vi "Calc Formation Energy from Defect Cluster.vi"(4 "Dielectric Constant":dbl=11.0, 6 "Volume (A³)":dbl=7795.605843681768, 8 "Markov-Payne Correction":bool, 9 "Chemical Potential":dbl(slide)=0.5124378109452736 scale=0.0..1.0, 10 "Fermi Level (eV)":dbl=1.8, 11 "Defect Data":T1={"Defect Details"={"Defect Name"="Cd Frenkel anion", "Site Density"=1.0, "Reference Pure Structure Energy"=-159.32149, "N (Cd,Ideal - Cd,Defect)"=0, "N (Te,ideal - Te,defect)"=0}, "Charges and Energies"=[]}) -> (2 "Net Charge":i32, 3 "Formation Energy (eV)":dbl)   [LabVIEW 2010]
panel:
  out "Array":dbl[](array[numeric])
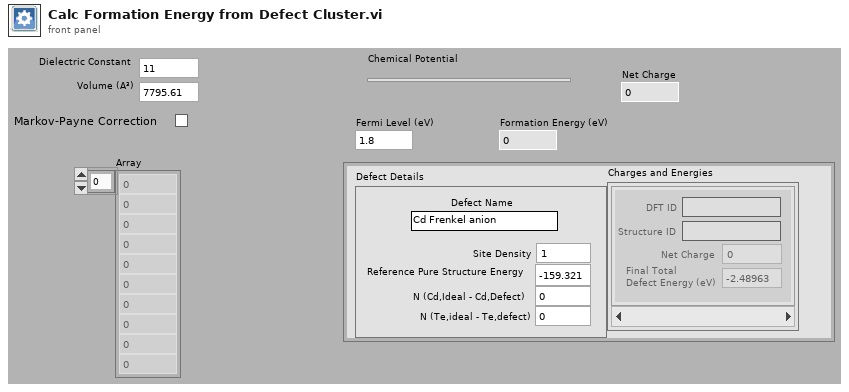
[diagram p1: front panel]
types:
  T1 = cluster{"Defect Details":cluster{"Defect Name":string, "Site Density":dbl, "Reference Pure Structure Energy":dbl, "N (Cd,Ideal - Cd,Defect)":i32, "N (Te,ideal - Te,defect)":i32}, "Charges and Energies":cluster{"DFT ID":string, "Structure ID":string, "Net Charge":i32, "Final Total \nDefect Energy (eV)":dbl}[]}
  T2 = cluster{"Defect Name":string, "Site Density":dbl, "Reference Pure Structure Energy":dbl, "N (Cd,Ideal - Cd,Defect)":i32, "N (Te,ideal - Te,defect)":i32}
  T3 = cluster{"DFT ID":string, "Structure ID":string, "Net Charge":i32, "Final Total \nDefect Energy (eV)":dbl}[]
  T4 = cluster{"DFT ID":string, "Structure ID":string, "Net Charge":i32, "Final Total \nDefect Energy (eV)":dbl}
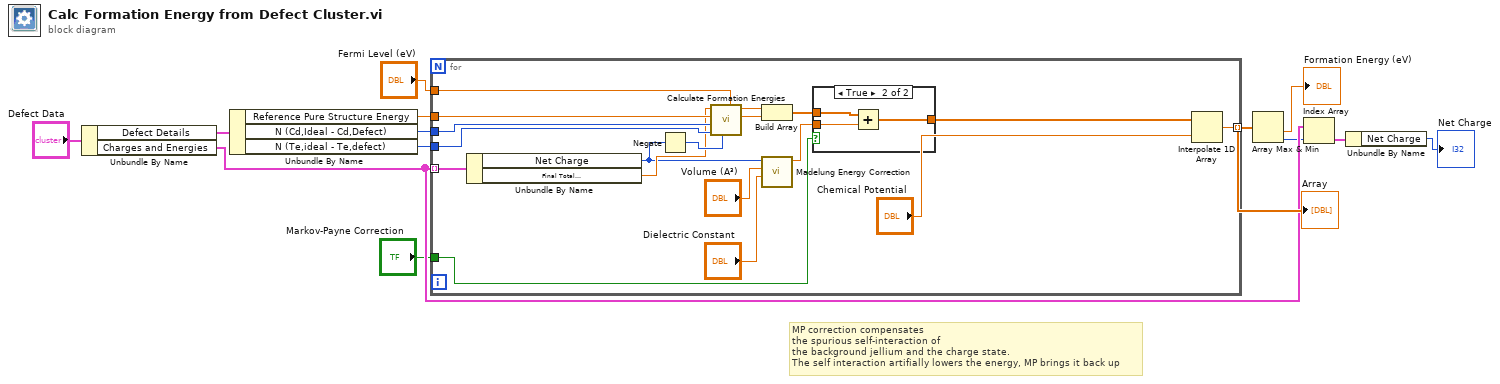
[diagram p0: block diagram]
diagram:
  # "MP correction compensates\nthe spurious self-interaction of\nthe background jellium and the charge state.\nThe self interaction artifially lowers the energy, MP brings it back up"
  n1 = Unbundle By Name("Defect Data") -> ("Defect Details"=w12:T2, "Charges and Energies"=w5:T3)
  n2 = Unbundle By Name(w12) -> ("Reference Pure Structure Energy"=w9:dbl, "N (Cd,Ideal - Cd,Defect)"=w11:i32, "N (Te,ideal - Te,defect)"=w10:i32)
  n3 = for {
    tunnel: [w21] -> w8 mode=indexing
    tunnel: "Fermi Level (eV)" -> [w31]
    tunnel: w11 -> [w30]
    tunnel: w10 -> [w29]
    tunnel: w9 -> [w28]
    tunnel: w5 -> [w27] mode=indexing
    tunnel: "Markov-Payne Correction" -> [w14]
    n4 = Unbundle By Name(w27) -> ("Net Charge"=w20:i32, "Final Total \nDefect Energy (eV)"=w25:dbl)
    n5 = Negate(x=w20) -> (-x=w26:i32)
    n6 = call "Calculate Formation Energies.vi"("Fermi (electron) energy (eV)"=w31, "# Extra Electrons"=w26, "N (Te,ideal - Te,defect)"=w29, "N (Cd,Ideal - Cd,Defect)"=w30, "Reference Pure Structure Energy"=w28, "Final Total Defect Energy (eV)"=w25) -> ("Formation Energy (Te-Rich)"=w23:dbl, "Formation Energy (Cd-Rich)"=w24:dbl)  [unwired: 4 in]
    n7 = Build Array(w24, w23) -> (w17:dbl[])
    n8 = call "Madelung Energy Correction.vi"("Dielectric Constant"="Dielectric Constant", "Volume (A³)"="Volume (A³)", "Net Charge"=w20) -> ("1st Order correction (eV)"=w16:dbl)  [unwired: 7 in, 1 out]
    n9 = case shown="True" w14 {
      tunnel: w17 -> [w32 w35]
      tunnel: w16 -> [_ w34]
      tunnel: [w32 w33] -> w15
      frame False {
      }
      frame True {
        n10 = Add(x=w35, y=w34) -> (x+y=w33:dbl[])
      }
    }
    n11 = Interpolate 1D Array(1:"Chemical Potential", 2:w15) -> (0:w21:dbl)
  }
  "Array" <- w8
  n12 = Array Max & Min(array=w8) -> (min value=→"Formation Energy (eV)":dbl, min index (indices)=w4:i32)  [unwired: 2 out]
  n13 = Index Array(array=w5, index=w4) -> (element=w3:T4)
  n14 = Unbundle By Name(w3) -> ("Net Charge"=→"Net Charge":i32)
